vi "GetProcessModeParamsFromDict.vi"(10 "Ink":T3[](array[typedef]), 11 "Data Value Reference in":T2) -> (2 "ProcessModeParams":T5)   [LabVIEW 2022 SP3, in "TopLevel.lvclass"]
uses:
  TopLevel.lvclass
  Typedefs/processMode_parameters--cluster.ctl
  DLP2/DataTypes/DLP2_PrinterMaterialProperties.ctl
  Typedefs/InkIdleNodeConfigXML--Cluster.ctl
  <vilib>/TELLC/Dynamic CVT API/TD Dynamic CVT DVR--ref.ctl
  Common/Controls/DLP_MaterialToHeadMapping--Cluster.ctl
  <userlib>/_OpenG.lib/array/array.llb/Sort 1D Array (U8)__ogtk.vi
  <userlib>/_OpenG.lib/array/array.llb/Reorder 1D Array2 (Boolean)__ogtk.vi
  <userlib>/_OpenG.lib/array/array.llb/Reorder 1D Array2 (DBL)__ogtk.vi
panel:
  in  "PrinterInitialization.HIBEnable.#attributes":T1
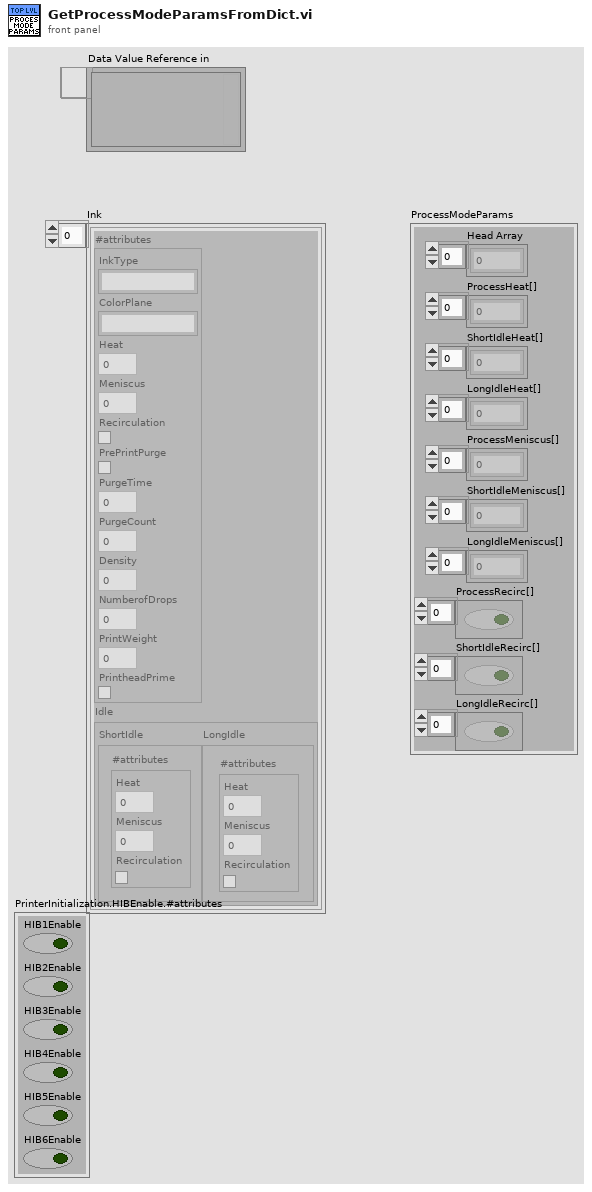
[diagram p1: front panel]
types:
  T1 = cluster{"HIB1Enable":bool, "HIB2Enable":bool, "HIB3Enable":bool, "HIB4Enable":bool, "HIB5Enable":bool, "HIB6Enable":bool}
  T2 = typedef "TD Dynamic CVT DVR--ref.ctl" = refnum<data-value>
  T3 = typedef "DLP2_PrinterMaterialProperties.ctl" = cluster{"#attributes":cluster{"InkType":string, "ColorPlane":string, "Heat":dbl, "Meniscus":dbl, "Recirculation":bool, "PrePrintPurge":bool, "PurgeTime":dbl, "PurgeCount":i32, "Density":dbl, "NumberofDrops":i32, "PrintWeight":dbl, "PrintheadPrime":bool}, "Idle":T4}
  T4 = typedef "InkIdleNodeConfigXML--Cluster.ctl" = cluster{"ShortIdle":cluster{"#attributes":cluster{"Heat":dbl, "Meniscus":dbl, "Recirculation":bool}}, "LongIdle":cluster{"#attributes":cluster{"Heat":dbl, "Meniscus":dbl, "Recirculation":bool}}}
  T5 = typedef "processMode_parameters--cluster.ctl" = cluster{"Head Array":u8[], "ProcessHeat[]":dbl[], "ShortIdleHeat[]":dbl[], "LongIdleHeat[]":dbl[], "ProcessMeniscus[]":dbl[], "ShortIdleMeniscus[]":dbl[], "LongIdleMeniscus[]":dbl[], "ProcessRecirc[]":bool[], "ShortIdleRecirc[]":bool[], "LongIdleRecirc[]":bool[]}
  T6 = typedef "DLP_MaterialToHeadMapping--Cluster.ctl" = cluster{"Head":u8, "Ink":T3}
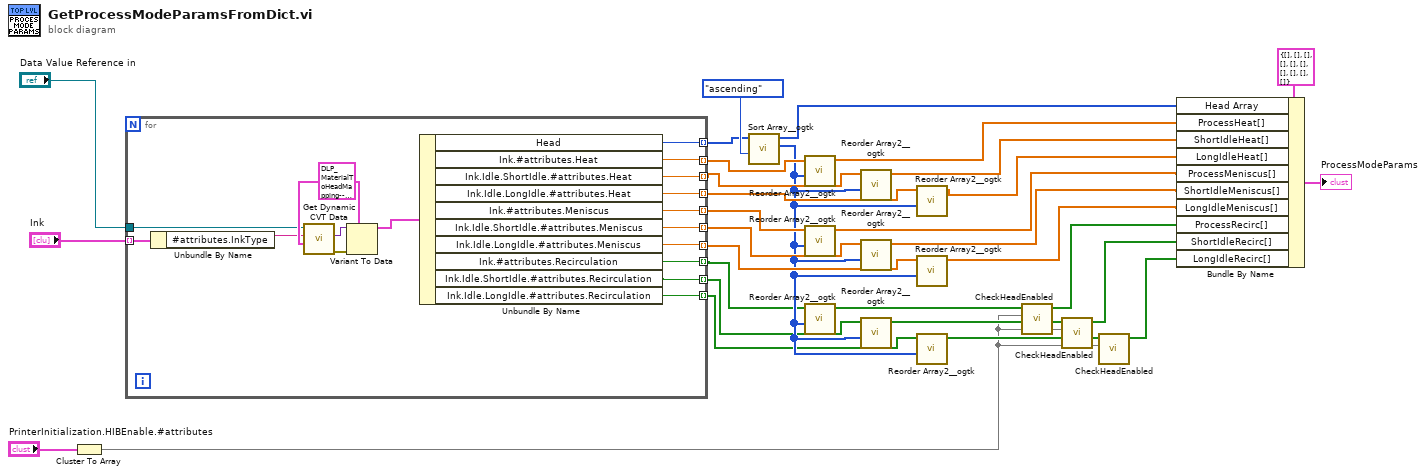
[diagram p0: block diagram]
diagram:
  n1 = Cluster To Array(cluster="PrinterInitialization.HIBEnable.#attributes") -> (array=w1:bool[])
  n2 = for {
    tunnel: "Data Value Reference in" -> [w44]
    tunnel: "Ink" -> [w43] mode=indexing
    tunnel: [w41] -> w21 mode=indexing
    tunnel: [w40] -> w23 mode=indexing
    tunnel: [w39] -> w24 mode=indexing
    tunnel: [w38] -> w25 mode=indexing
    tunnel: [w37] -> w18 mode=indexing
    tunnel: [w36] -> w17 mode=indexing
    tunnel: [w35] -> w16 mode=indexing
    tunnel: [w34] -> w11 mode=indexing
    tunnel: [w33] -> w10 mode=indexing
    tunnel: [w32] -> w9 mode=indexing
    w46 = T6 {"Head"=0, "Ink"={"#attributes"={"InkType"="", "ColorPlane"="", "Heat"=0.0, "Meniscus"=0.0, "Recirculation"=FALSE, "PrePrintPurge"=FALSE, "PurgeTime"=0.0, "PurgeCount"=0, "Density"=0.0, "NumberofDrops"=0, "PrintWeight"=0.0, "PrintheadPrime"=FALSE}, "Idle"={"ShortIdle"={"#attributes"={"Heat"=0.0, "Meniscus"=0.0, "Recirculation"=FALSE}}, "LongIdle"={"#attributes"={"Heat"=0.0, "Meniscus"=0.0, "Recirculation"=FALSE}}}}}
    n3 = Unbundle By Name(w43) -> ("#attributes.InkType"=w42:string)
    n4 = call <vilib>:"Get Dynamic CVT Data.vi"("default value (empty variant)"=w46, "DataName"=w42, "dCVT DVR"=w44) -> ("error out"=w48:errorcluster, "value"=w47:variant)  [unwired: 5 in, 2 out]
    n5 = Variant To Data(error in=w48, type=w46, Variant=w47) -> (data=w45:T6)  [unwired: 1 out]
    n6 = Unbundle By Name(w45) -> ("Head"=w41:u8, "Ink.#attributes.Heat"=w40:dbl, "Ink.Idle.ShortIdle.#attributes.Heat"=w39:dbl, "Ink.Idle.LongIdle.#attributes.Heat"=w38:dbl, "Ink.#attributes.Meniscus"=w37:dbl, "Ink.Idle.ShortIdle.#attributes.Meniscus"=w36:dbl, "Ink.Idle.LongIdle.#attributes.Meniscus"=w35:dbl, "Ink.#attributes.Recirculation"=w34:bool, "Ink.Idle.ShortIdle.#attributes.Recirculation"=w33:bool, "Ink.Idle.LongIdle.#attributes.Recirculation"=w32:bool)
  }
  n7 = call-poly <userlib>:"Sort Array__ogtk.vi"("Order"=enum16{"ascending", "descending"}."ascending", "Array in"=w21) -> ("Sorted Pointers"=w12:i32[], "Sorted Array out"=w27:u8[])  [unwired: 8 in]
  n8 = call-poly <userlib>:"Reorder Array2__ogtk.vi"("indices"=w12, "array"=w23) -> ("reordered array"=w28:dbl[])  [unwired: 9 in]
  n9 = call-poly <userlib>:"Reorder Array2__ogtk.vi"("indices"=w12, "array"=w18) -> ("reordered array"=w15:dbl[])  [unwired: 9 in]
  n10 = call-poly <userlib>:"Reorder Array2__ogtk.vi"("indices"=w12, "array"=w11) -> ("reordered array"=w7:bool[])  [unwired: 9 in]
  n11 = call-poly <userlib>:"Reorder Array2__ogtk.vi"("indices"=w12, "array"=w24) -> ("reordered array"=w29:dbl[])  [unwired: 9 in]
  n12 = call-poly <userlib>:"Reorder Array2__ogtk.vi"("indices"=w12, "array"=w17) -> ("reordered array"=w14:dbl[])  [unwired: 9 in]
  n13 = call-poly <userlib>:"Reorder Array2__ogtk.vi"("indices"=w12, "array"=w10) -> ("reordered array"=w3:bool[])  [unwired: 9 in]
  n14 = call-poly <userlib>:"Reorder Array2__ogtk.vi"("indices"=w12, "array"=w25) -> ("reordered array"=w31:dbl[])  [unwired: 9 in]
  n15 = call-poly <userlib>:"Reorder Array2__ogtk.vi"("indices"=w12, "array"=w16) -> ("reordered array"=w13:dbl[])  [unwired: 9 in]
  n16 = call-poly <userlib>:"Reorder Array2__ogtk.vi"("indices"=w12, "array"=w9) -> ("reordered array"=w5:bool[])  [unwired: 9 in]
  n17 = call "CheckHeadEnabled.vi"("PrinterInitialization.HIBEnable.#attributes"=w1, "reordered array"=w7) -> ("Array"=w6:bool[])  [unwired: 9 in]
  n18 = call "CheckHeadEnabled.vi"("PrinterInitialization.HIBEnable.#attributes"=w1, "reordered array"=w3) -> ("Array"=w2:bool[])  [unwired: 9 in]
  n19 = call "CheckHeadEnabled.vi"("PrinterInitialization.HIBEnable.#attributes"=w1, "reordered array"=w5) -> ("Array"=w4:bool[])  [unwired: 9 in]
  n20 = Bundle By Name(cluster=T5 {"Head Array"=[], "ProcessHeat[]"=[], "ShortIdleHeat[]"=[], "LongIdleHeat[]"=[], "ProcessMeniscus[]"=[], "ShortIdleMeniscus[]"=[], "LongIdleMeniscus[]"=[], "ProcessRecirc[]"=[], "ShortIdleRecirc[]"=[], "LongIdleRecirc[]"=[]}, "Head Array"=w27, "ProcessHeat[]"=w28, "ShortIdleHeat[]"=w29, "LongIdleHeat[]"=w31, "ProcessMeniscus[]"=w15, "ShortIdleMeniscus[]"=w14, "LongIdleMeniscus[]"=w13, "ProcessRecirc[]"=w6, "ShortIdleRecirc[]"=w2, "LongIdleRecirc[]"=w4) -> (→"ProcessModeParams":T5)
